vi "REST Client - VI Tree.vi"   [LabVIEW 2020]
uses:
  classes/REST Client/REST Client.lvclass
  classes/Response Headers/Response Headers.lvclass
  classes/http-client/http-client.lvclass
  classes/REST Client/HTTP Header.ctl
  classes/REST Client/HTTP Methods.ctl
types:
  T1 = typedef "REST Client.lvlib/REST Client.lvclass/HTTP Methods.ctl" = enum16{"GET", "HEAD", "POST", "PUT", "DELETE", "PATCH"}
  T2 = typedef "REST Client.lvlib/REST Client.lvclass/HTTP Header.ctl" = cluster{"header":string, "value":string}
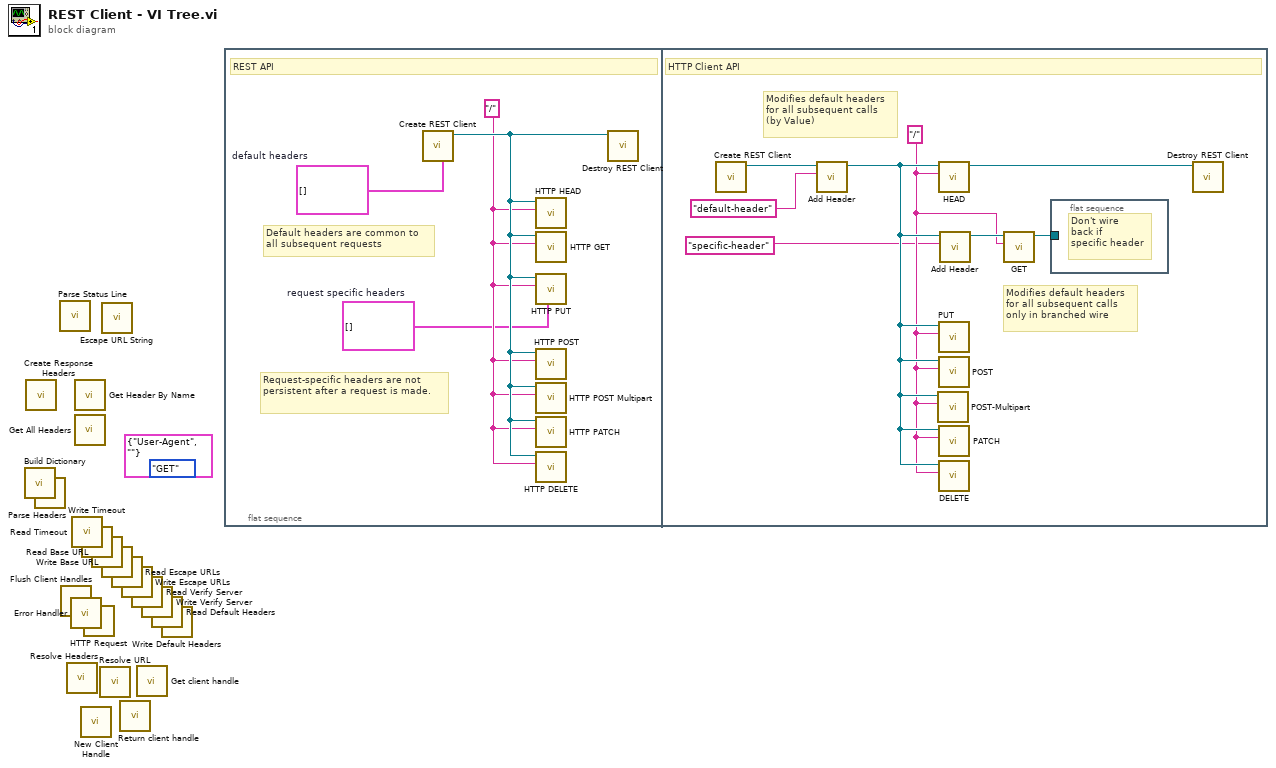
[diagram p0: block diagram]
diagram:
  (unwired) HTTP_Methods."GET" ("HTTP method")
  (unwired) T2 {"header"="User-Agent", "value"=""} ("Header")
  n1 = call "Build Dictionary.vi"() -> ()  [unwired: 10 in, 2 out]
  n2 = call "Create Response Headers.vi"() -> ()  [unwired: 10 in, 2 out]
  n3 = call "Parse Headers.vi"() -> ()  [unwired: 11 in, 1 out]
  n4 = call "Parse Status Line.vi"() -> ()  [unwired: 7 in, 5 out]
  n5 = call-dynamic "Flush Client Handles.vi"() -> ()  [unwired: 10 in, 2 out]
  n6 = call "Resolve Headers.vi"() -> ()  [unwired: 11 in, 1 out]
  n7 = call-dynamic "Error Handler.vi"() -> ()  [unwired: 10 in, 2 out]
  n8 = call-dynamic "Read Timeout.vi"() -> ()  [unwired: 9 in, 3 out]
  n9 = call "Get Header By Name.vi"() -> ()  [unwired: 8 in, 4 out]
  n10 = call "Get All Headers.vi"() -> ()  [unwired: 8 in, 4 out]
  n11 = call "New Client Handle.vi"() -> ()  [unwired: 9 in, 3 out]
  n12 = call-dynamic "Write Timeout.vi"() -> ()  [unwired: 10 in, 2 out]
  n13 = call-dynamic "HTTP Request.vi"() -> ()  [unwired: 10 in, 6 out]
  n14 = call-dynamic "Read Base URL.vi"() -> ()  [unwired: 9 in, 3 out]
  n15 = call "Resolve URL.vi"() -> ()  [unwired: 11 in, 1 out]
  n16 = call "Escape URL String.vi"() -> ()  [unwired: 1 in, 1 out]
  n17 = call-dynamic "Write Base URL.vi"() -> ()  [unwired: 10 in, 2 out]
  n18 = call-dynamic "Read Escape URLs.vi"() -> ()  [unwired: 9 in, 3 out]
  n19 = call "Return client handle.vi"() -> ()  [unwired: 10 in, 2 out]
  n20 = call-dynamic "Write Escape URLs.vi"() -> ()  [unwired: 10 in, 2 out]
  n21 = call-dynamic "Read Verify Server.vi"() -> ()  [unwired: 9 in, 3 out]
  n22 = call "Get client handle.vi"() -> ()  [unwired: 8 in, 4 out]
  n23 = call-dynamic "Write Verify Server.vi"() -> ()  [unwired: 10 in, 2 out]
  n24 = call-dynamic "Read Default Headers.vi"() -> ()  [unwired: 9 in, 3 out]
  n25 = call-dynamic "Write Default Headers.vi"() -> ()  [unwired: 10 in, 2 out]
  n26 = flat-sequence {
    frame #0 {
      w2 = T2[] []  # default headers
      w1 = T2[] []  # request specific headers
      w3 = "/" ("url")
      # "Default headers are common to\nall subsequent requests"
      # "Request-specific headers are not persistent after a request is made."
      # "REST API"
      n27 = call "Create REST Client.vi"("Default Headers ([JSON])"=w2) -> ("REST Client out"=w4:refnum<class "REST Client.lvclass">)  [unwired: 9 in, 1 out]
      n28 = call-dynamic "HTTP HEAD.vi"("Path"=w3, "REST Client in"=w4) -> ()  [unwired: 4 in, 6 out]
      n29 = call-dynamic "HTTP GET.vi"("Path"=w3, "REST Client in"=w4) -> ()  [unwired: 4 in, 6 out]
      n30 = call-dynamic "HTTP PUT.vi"("request specific headers"=w1, "Path"=w3, "REST Client in"=w4) -> ()  [unwired: 3 in, 6 out]
      n31 = call-dynamic "HTTP POST.vi"("Path"=w3, "REST Client in"=w4) -> ()  [unwired: 4 in, 6 out]
      n32 = call-dynamic "HTTP POST Multipart.vi"("Path"=w3, "REST Client in"=w4) -> ()  [unwired: 4 in, 6 out]
      n33 = call-dynamic "HTTP PATCH.vi"("Path"=w3, "REST Client in"=w4) -> ()  [unwired: 4 in, 6 out]
      n34 = call-dynamic "HTTP DELETE.vi"("Path"=w3, "REST Client in"=w4) -> ()  [unwired: 4 in, 6 out]
      n35 = call-dynamic "Destroy REST Client.vi"("REST Client in"=w4) -> ()  [unwired: 10 in, 1 out]
    }
    frame #1 {
      w9 = "/" ("url")
      # "Modifies default headers\nfor all subsequent calls\nonly in branched wire"
      # "Modifies default headers\nfor all subsequent calls\n(by Value)"
      # "HTTP Client API"
      n36 = call "Create REST Client.vi"() -> ("REST Client out"=w12:refnum<class "REST Client.lvclass">)  [unwired: 10 in, 1 out]
      n37 = call "Add Header.vi"("header"="default-header" ("url"), "http-client in"=w12) -> ("http-client out"=w10:refnum<class "http-client.lvclass">)  [unwired: 8 in, 1 out]
      n38 = call "POST-Multipart.vi"("url"=w9, "http-client in"=w10) -> ()  [unwired: 5 in, 5 out]
      n39 = call "HEAD.vi"("url"=w9, "http-client in"=w10) -> ("http-client out"=w6:refnum<class "http-client.lvclass">)  [unwired: 6 in, 3 out]
      n40 = call "PUT.vi"("url"=w9, "http-client in"=w10) -> ()  [unwired: 5 in, 5 out]
      n41 = call "POST.vi"("url"=w9, "http-client in"=w10) -> ()  [unwired: 5 in, 5 out]
      n42 = call "PATCH.vi"("url"=w9, "http-client in"=w10) -> ()  [unwired: 5 in, 5 out]
      n43 = call "DELETE.vi"("url"=w9, "http-client in"=w10) -> ()  [unwired: 5 in, 5 out]
      n44 = call "Add Header.vi"("header"="specific-header" ("url"), "http-client in"=w10) -> ("http-client out"=w11:refnum<class "http-client.lvclass">)  [unwired: 8 in, 1 out]
      n45 = call "GET.vi"("url"=w9, "http-client in"=w11) -> ("http-client out"=w5:refnum<class "http-client.lvclass">)  [unwired: 5 in, 4 out]
      n46 = flat-sequence {
        tunnel: w5 -> [_]
        frame #0 {
          # "Don't wire\nback if\nspecific header"
        }
      }
      n47 = call-dynamic "Destroy REST Client.vi"("REST Client in"=w6) -> ()  [unwired: 10 in, 1 out]
    }
  }
